vi "Read TxPkt Loop Period.vi"(8 "error in (no error)":errorcluster, 11 "Node Ptr":T1 format="%.0x") -> (0 "error out":errorcluster, 2 "loopPeriod":u32=1 caption="Loop Period (us)" min=1 step=1, 3 "Node Ptr out":T1 format="%.0x")   [LabVIEW 2016, in "UDP-Custom-Device System Explorer.lvlib" / "Tx Packet Accessors.lvlib"]
uses:
  Tx Packet Accessors.lvlib
  <vilib>/NI Veristand/Custom Device API/Custom Device Item Ref.ctl
  <vilib>/NI Veristand/Custom Device API/Custom Device Target Type.ctl
  Shared/Constants.vi
  <vilib>/NI Veristand/Custom Device API/Get Item Property (I32).vi
  <vilib>/NI VeriStand/Custom Device API/Custom Device API.lvlib
  Shared/UDP-Custom-Device Shared.lvlib
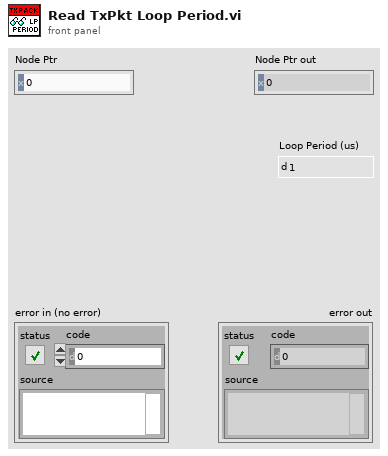
[diagram p1: front panel]
types:
  T1 = typedef "Custom Device API.lvlib/Custom Device Item Ref.ctl" = u64
  T2 = typedef "Custom Device API.lvlib/Custom Device Target Type.ctl" = enum16{"PharLap", "VxWorks", "Windows", "Linux_32_ARM", "Linux_x64"}
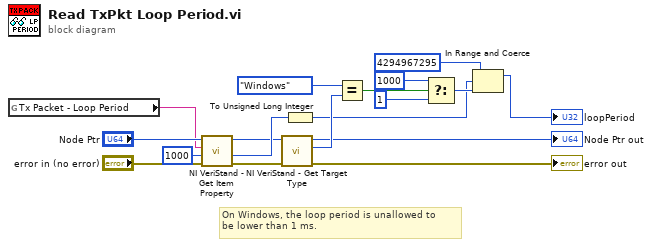
[diagram p0: block diagram]
diagram:
  # "On Windows, the loop period is unallowed to\nbe lower than 1 ms."
  n1 = global read "Constants.vi" "Tx Packet - Loop Period"() -> (w14:string)
  n2 = call-poly <vilib>:"NI VeriStand - Get Item Property.vi"("error in (no error)"="error in (no error)", "Default Value"=1000, "Property Name"=w14, "Item Ref in"="Node Ptr") -> ("error out"=w6:errorcluster, "Value"=w16:i32, "Item Ref out"=w4:T1)  [unwired: 4 in, 1 out]
  n3 = call <vilib>:"NI VeriStand - Get Target Type.vi"("error in (no error)"=w6, "Item Ref in"=w4) -> ("error out"=→"error out":errorcluster, "Target Type"=w12:T2, "Item Ref out"=→"Node Ptr out":T1)  [unwired: 7 in]
  n4 = To Unsigned Long Integer(number=w16) -> (unsigned 32bit integer=w2:u32)
  n5 = Equal?(x=Custom_Device_Target_Type."Windows" ("y"), y=w12) -> (x = y?=w9:bool)
  n6 = Select(t=u32 1000 ("lower limit"), s=w9, f=u32 1 ("lower limit")) -> (s? t:f=w8:u32)
  n7 = In Range and Coerce(upper limit=u32 4294967295 ("loopPeriod"), x=w2, lower limit=w8) -> (coerced(x)=→"loopPeriod":u32)  [unwired: 1 out]
